vi "Triangulate Spark LLS.vi"(3 "Sensor Errors (s)":dbl[](array[numeric])=[0.01639, 0.01306, 0.01306, 0.01306, 0.01306, 0.01639], 4 "Sensor Locations (m)":dbl[][](array[numeric])=[[0.0, 0.0, -0.04048], [0.1143, 0.0, 0.0], [0.0, 0.1143, 0.0], [-0.1143, 0.0, 0.0], [0.0, -0.1143, 0.0], [0.0, 0.0, 0.04048]], 5 "Wavefront Times (s)":dbl[](array[numeric])) -> (0 "X with Errors":cluster{"x":dbl, "y":dbl, "z":dbl}, 1 "X":cluster{"x":dbl, "y":dbl, "z":dbl})   [LabVIEW 2013]
uses:
  <vilib>/Analysis/Matrix/Datatypes/RealMatrix.ctl
  <vilib>/Analysis/baseanly.llb/Real A x B.vi
  <vilib>/Analysis/baseanly.llb/A x Vector.vi
  <vilib>/Analysis/baseanly.llb/Real Inverse Matrix.vi
  <vilib>/Analysis/Matrix/Numeric/Conversions/Array To Matrix - RA2.vi
  <vilib>/Analysis/Matrix/NI_Matrix.lvlib
  <vilib>/Analysis/NI_AALBase.lvlib
panel:
  out "Spark Radii (m)":dbl[](array[numeric])
  out "error":i32
  out "W":T1
  out "Q":T1
  out "B":T1
  out "b":dbl[](array[numeric])
  out "(A^T A)^(-1) A^T":T1
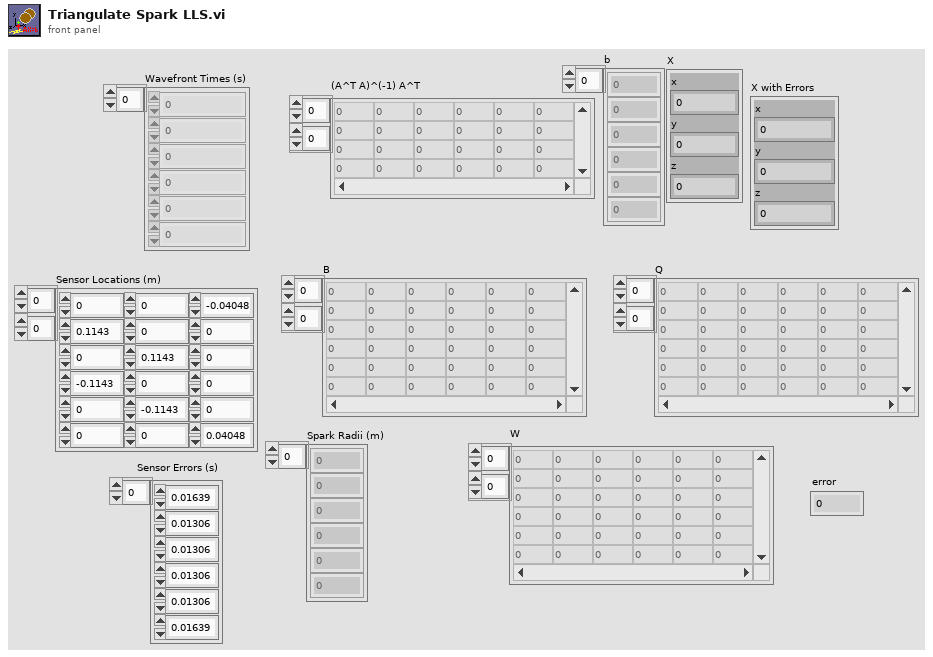
[diagram p1: front panel]
types:
  T1 = typedef "NI_Matrix.lvlib/RealMatrix.ctl" = dbl[][]
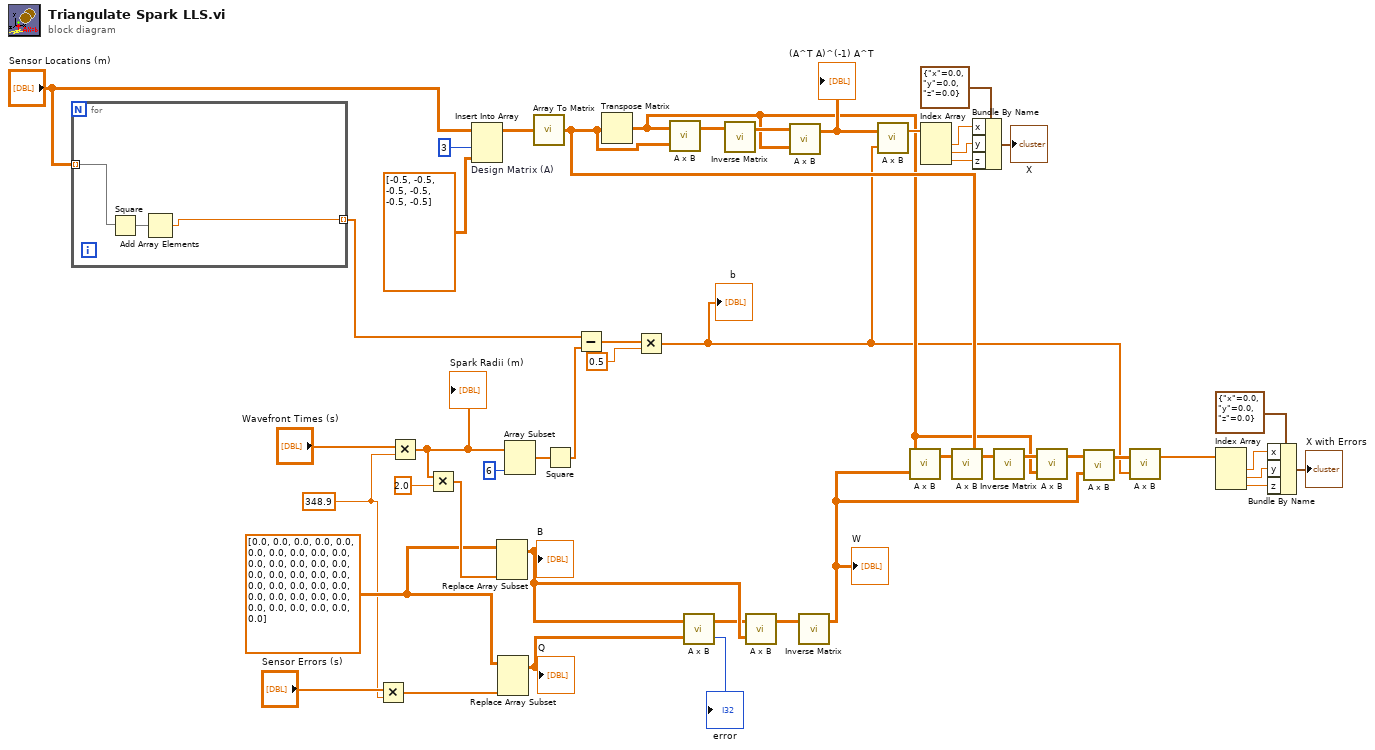
[diagram p0: block diagram]
diagram:
  w36 = T1 [[0.0, 0.0, 0.0, 0.0, 0.0, 0.0], [0.0, 0.0, 0.0, 0.0, 0.0, 0.0], [0.0, 0.0, 0.0, 0.0, 0.0, 0.0], [0.0, 0.0, 0.0, 0.0, 0.0, 0.0], [0.0, 0.0, 0.0, 0.0, 0.0, 0.0], [0.0, 0.0, 0.0, 0.0, 0.0, 0.0]] ("matrix")
  w6 = 348.9
  n1 = for {
    tunnel: "Sensor Locations (m)" -> [w48] mode=indexing
    tunnel: [w49] -> w1 mode=indexing
    n2 = Square(x=w48) -> (x^2=w50:dbl[])
    n3 = Add Array Elements(numeric array=w50) -> (sum=w49:dbl)
  }
  n4 = Multiply(x="Sensor Errors (s)", y=w6) -> (x*y=w29:dbl[])
  n5 = Multiply(x="Wavefront Times (s)", y=w6) -> (x*y=w39:dbl[])
  "Spark Radii (m)" <- w39
  n6 = Multiply(x=w39, y=2.0) -> (x*y=w37:dbl[])
  n7 = Insert Into Array "Design Matrix (A)"(array="Sensor Locations (m)", index (col)=3 ("disabled index (col)"), new element=dbl[][] [[-0.5], [-0.5], [-0.5], [-0.5], [-0.5], [-0.5]] ("Real 2D Array")) -> (w3:dbl[][])  [unwired: 1 in]
  n8 = Replace Array Subset(array=w36, new element=w37) -> (w34:T1)  [unwired: 2 in]
  "B" <- w34
  n9 = Replace Array Subset(array=w36, new element=w29) -> (w35:T1)  [unwired: 2 in]
  "Q" <- w35
  n10 = Array Subset(array=w39, length=6) -> (w46:dbl[])  [unwired: 1 in]
  n11 = call-poly <vilib>:"Array To Matrix.vi"("Real 2D Array"=w3) -> ("Real Matrix"=w16:T1)
  n12 = Square(x=w46) -> (x^2=w45:dbl[])
  n13 = Subtract(x=w1, y=w45) -> (x-y=w41:dbl[])
  n14 = Transpose Matrix(1:w16) -> (0:w12:T1)
  n15 = Multiply(x=w41, y=0.5) -> (x*y=w8:dbl[])
  "b" <- w8
  n16 = call-poly <vilib>:"A x B.vi"("B"=w16, "A"=w12) -> ("A x B"=w44:T1)  [unwired: 1 out]
  n17 = call-poly <vilib>:"A x B.vi"("B"=w35, "A"=w34) -> ("error"=→"error":i32, "A x B"=w32:T1)
  n18 = call-poly <vilib>:"Inverse Matrix.vi"("Input Matrix"=w44) -> ("Inverse Matrix"=w43:T1)  [unwired: 1 in, 1 out]
  n19 = call-poly <vilib>:"A x B.vi"("B"=w34, "A"=w32) -> ("A x B"=w33:T1)  [unwired: 1 out]
  n20 = call-poly <vilib>:"A x B.vi"("B"=w12, "A"=w43) -> ("A x B"=w28:T1)  [unwired: 1 out]
  "(A^T A)^(-1) A^T" <- w28
  n21 = call-poly <vilib>:"Inverse Matrix.vi"("Input Matrix"=w33) -> ("Inverse Matrix"=w10:T1)  [unwired: 1 in, 1 out]
  "W" <- w10
  n22 = call-poly <vilib>:"A x B.vi"("Vector"=w8, "A"=w28) -> ("A x Vector"=w27:dbl[])  [unwired: 1 out]
  n23 = call-poly <vilib>:"A x B.vi"("B"=w10, "A"=w12) -> ("A x B"=w15:T1)  [unwired: 1 out]
  n24 = Index Array(array=w27) -> (element #1=w25:dbl, element #2=w24:dbl, element #3=w23:dbl)  [unwired: 3 in]
  n25 = call-poly <vilib>:"A x B.vi"("B"=w16, "A"=w15) -> ("A x B"=w14:T1)  [unwired: 1 out]
  n26 = Bundle By Name(cluster=cluster{"x":dbl, "y":dbl, "z":dbl} {"x"=0.0, "y"=0.0, "z"=0.0} ("input cluster"), "x"=w25, "y"=w24, "z"=w23) -> (→"X":cluster{"x":dbl, "y":dbl, "z":dbl})
  n27 = call-poly <vilib>:"Inverse Matrix.vi"("Input Matrix"=w14) -> ("Inverse Matrix"=w13:T1)  [unwired: 1 in, 1 out]
  n28 = call-poly <vilib>:"A x B.vi"("B"=w12, "A"=w13) -> ("A x B"=w11:T1)  [unwired: 1 out]
  n29 = call-poly <vilib>:"A x B.vi"("B"=w10, "A"=w11) -> ("A x B"=w9:T1)  [unwired: 1 out]
  n30 = call-poly <vilib>:"A x B.vi"("Vector"=w8, "A"=w9) -> ("A x Vector"=w7:dbl[])  [unwired: 1 out]
  n31 = Index Array(array=w7) -> (element #1=w20:dbl, element #2=w19:dbl, element #3=w18:dbl)  [unwired: 3 in]
  n32 = Bundle By Name(cluster=cluster{"x":dbl, "y":dbl, "z":dbl} {"x"=0.0, "y"=0.0, "z"=0.0} ("input cluster"), "x"=w20, "y"=w19, "z"=w18) -> (→"X with Errors":cluster{"x":dbl, "y":dbl, "z":dbl})
